vi "Configure RemIO Module.vi"(8 "error in (no error)":errorcluster, 9 "Slave Ref In":refnum<k21>, 10 "RemIO Module in":refnum<class "RemIO Module.lvclass">, 11 "Node Ptr In":T1 format="%.0x") -> (0 "error out":errorcluster, 1 "Slave Ref Out":refnum<k21>, 2 "RemIO Module out":refnum<class "RemIO Module.lvclass">, 3 "Node Ptr Out":T1 format="%.0x")   [LabVIEW 2019, in "Modules.lvlib" / "RemIO Module.lvclass"]
uses:
  RemIO Module.lvclass
  <vilib>/NI VeriStand/Custom Device API/Custom Device Item Ref.ctl
  <vilib>/Utility/error.llb/Error Cluster From Error Code.vi
  <vilib>/ErrorRing/Error Ring.xnode
  <vilib>/NI VeriStand/Custom Device API/Custom Device API.lvlib
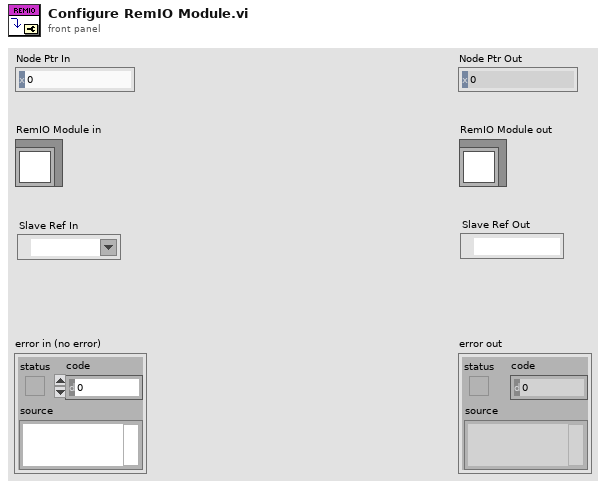
[diagram p1: front panel]
types:
  T1 = typedef "Custom Device API.lvlib/Custom Device Item Ref.ctl" = u64
  T2 = typedef "negative confirmation.ctl" = cluster{"error code":u16, "additional error code":u16}
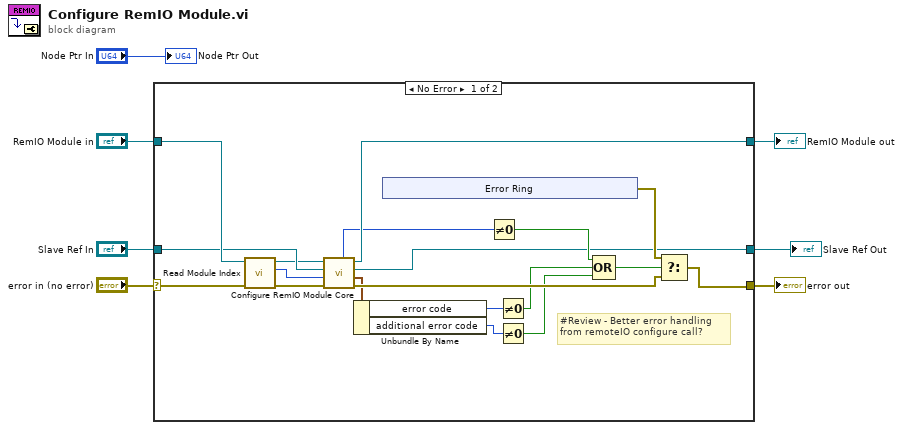
[diagram p0: block diagram]
diagram:
  n1 = case shown="No Error" "error in (no error)" {
    selector: "error in (no error)" -> [w24 w34]
    tunnel: [w25 w34] -> w6
    tunnel: [w14 w33] -> w4
    tunnel: "RemIO Module in" -> [w23 w33]
    tunnel: [w16 w32] -> w3
    tunnel: "Slave Ref In" -> [w18 w32]
    frame No Error {
      # "#Review - Better error handling\nfrom remoteIO configure call?"
      n2 = call-dynamic "Read Module Index.vi"("error in (no error)"=w24, "RemIO Module in"=w23) -> ("error out"=w20:errorcluster, "Module Index"=w17:u8, "RemIO Module out"=w15:refnum<class "RemIO Module.lvclass">)  [unwired: 7 in]
      n3 = call-dynamic "Configure RemIO Module Core.vi"("error in (no error)"=w20, "module slot index"=w17, "Slave Ref In"=w18, "RemIO Module in"=w15) -> ("error out"=w19:errorcluster, "negative confirmation"=w12:T2, "Slave Ref Out"=w16:refnum<k21>, "RemIO Module out"=w14:refnum<class "RemIO Module.lvclass">, "SDO abort code"=w13:u32)  [unwired: 3 in]
      n4 = Unbundle By Name(w12) -> ("error code"=w10:u16, "additional error code"=w11:u16)
      n5 = xnode "Error Ring"() -> ("error out"=w26:errorcluster)
      n6 = Not Equal To 0?(x=w13) -> (x != 0?=w21:bool)
      n7 = Not Equal To 0?(x=w10) -> (x != 0?=w9:bool)
      n8 = Not Equal To 0?(x=w11) -> (x != 0?=w8:bool)
      n9 = Compound Arithmetic op=OR(w21, w9, w8) -> (w22:bool)
      n10 = Select(t=w26, s=w22, f=w19) -> (s? t:f=w25:errorcluster)
    }
    frame Error {
    }
  }
  "error out" <- w6
  "RemIO Module out" <- w4
  "Slave Ref Out" <- w3
  "Node Ptr Out" <- "Node Ptr In"
